vi "Get Source Auto Delay State.vi"(8 "error in (no error)":errorcluster, 10 "Function (0: Volts)":u16(ring) items=["Volts", "Current"], 11 "VISA resource name":refnum<visa-resource-name>) -> (0 "error out":errorcluster, 2 "Auto Delay Enabled?":bool, 3 "VISA resource name out":refnum<visa-resource-name>)   [LabVIEW 2017, in "Keithley 2450.lvlib"]
doc: "ThisVi returns whether the source autodelay is on or off for the selected source function."
uses:
  Keithley 2450.lvlib
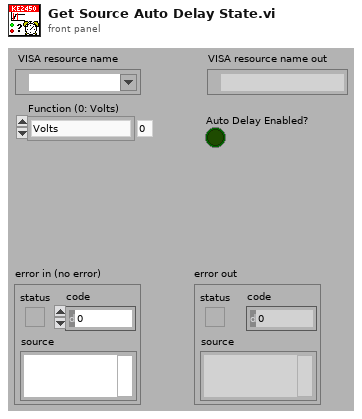
[diagram p1: front panel]
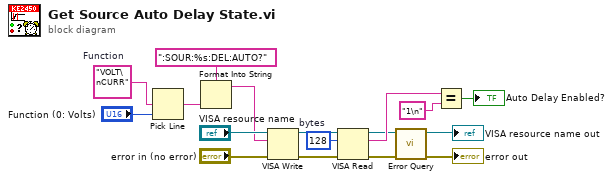
[diagram p0: block diagram]
diagram:
  w5 = u32 128  # bytes
  w11 = "VOLT\nCURR"  # Function
  n1 = Pick Line(multi-line string=w11, line index="Function (0: Volts)") -> (output string=w9:string)  [unwired: 1 out]
  n2 = Format Into String(format string=":SOUR:%s:DEL:AUTO?", w9) -> (resulting string=w12:string)  [unwired: 2 in, 1 out]
  n3 = VISA Write(VISA resource name="VISA resource name", write buffer=w12, error in (no error)="error in (no error)") -> (VISA resource name out=w4:refnum<visa-resource-name>, error out=w2:errorcluster)  [unwired: 1 out]
  n4 = VISA Read(VISA resource name=w4, byte count=w5, error in (no error)=w2) -> (VISA resource name out=w3:refnum<visa-resource-name>, read buffer=w8:string, error out=w1:errorcluster)  [unwired: 1 out]
  n5 = call "Error Query.vi"("error in (no error)"=w1, "VISA resource name"=w3) -> ("error out"=→"error out":errorcluster, "VISA resource name out"=→"VISA resource name out":refnum<visa-resource-name>)  [unwired: 8 out]
  n6 = Equal?(x=w8, y="1\n") -> (x = y?=→"Auto Delay Enabled?":bool)
